vi "Get Active Statement Function.vi"(0 "Statement in":refnum<class "Statement.lvclass">, 11 "error in (no error)":errorcluster) -> (4 "Statement out":refnum<class "Statement.lvclass">, 6 "Function List":T1, 15 "error out":errorcluster)   [LabVIEW 2016, in "Statement.lvclass"]
uses:
  Statement.lvclass
  E:/Repository/LabVIEW Script Language/source code/LSL components/functions/functionsbase/functionbase.lvclass
  Function List.ctl
  functionsbase/functionbase.lvclass
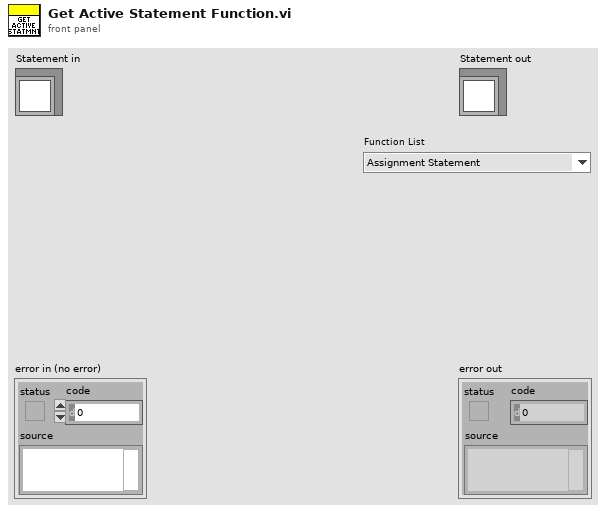
[diagram p1: front panel]
types:
  T1 = typedef "Statement.lvclass/Function List.ctl" = enum16{"Assignment Statement", "Comma Statement"}
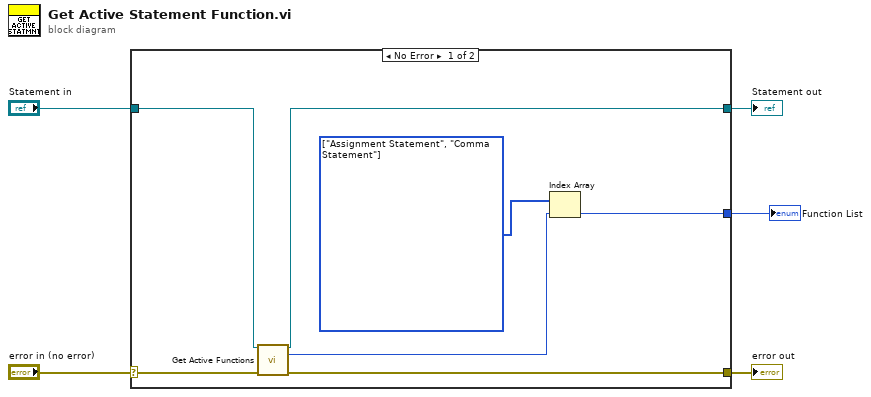
[diagram p0: block diagram]
diagram:
  n1 = case shown="No Error" "error in (no error)" {
    selector: "error in (no error)" -> [w12 w14]
    tunnel: [w11 w14] -> w4
    tunnel: [w9 w13] -> w2
    tunnel: "Statement in" -> [w10 w13]
    tunnel: [w6 _] -> w1
    frame No Error {
      w7 = T1[] [enum."Assignment Statement", enum."Comma Statement"] items=["Assignment Statement", "Comma Statement"]
      n2 = call "Get Active Functions.vi"("functionbase in"=w10, "error in (no error)"=w12) -> ("functionbase out"=w9:refnum<class "Statement.lvclass">, "Syntax Index"=w8:i32, "error out"=w11:errorcluster)  [unwired: 11 in]
      n3 = Index Array(array=w7, index=w8) -> (element=w6:T1)
    }
    frame Error {
    }
  }
  "error out" <- w4
  "Statement out" <- w2
  "Function List" <- w1
